vi "test_csm_interface_descp.vi"() -> ()   [LabVIEW 2020]
uses:
  Typedef/Def-Argument Info.ctl
  Create From VI Reference.vi
  Properties/Read User-Defined States.vi
  CSM-Helper.lvclass
panel:
  out "error out":errorcluster
  out "Array 3":cluster{string, "Argument":T1, "Response":T1}[](array[cluster])
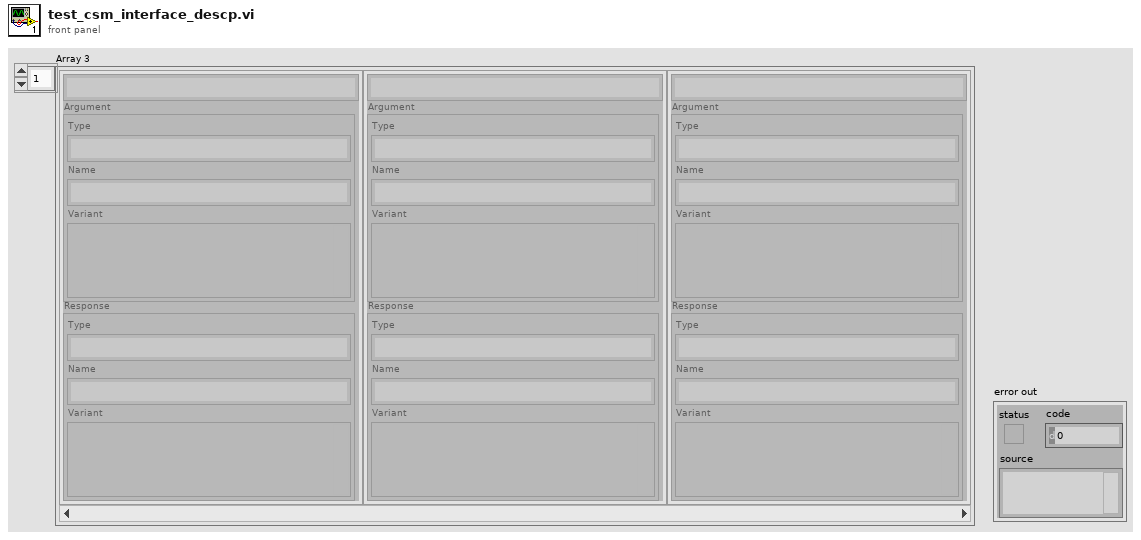
[diagram p1: front panel]
types:
  T1 = typedef "CSM-Helper.lvclass/Def-Argument Info.ctl" = cluster{"Type":string, "Name":string, "Variant":variant}
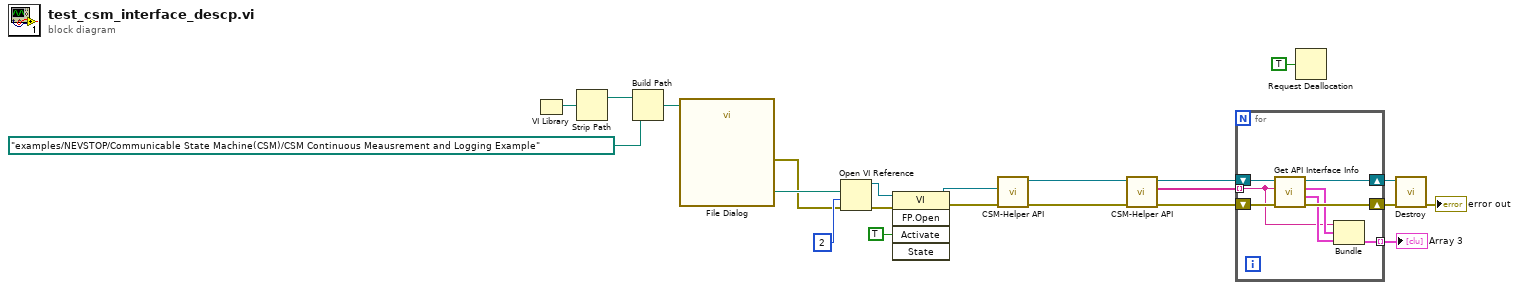
[diagram p0: block diagram]
diagram:
  n1 = VI Library() -> (path=w22:path)
  n2 = Strip Path(path=w22) -> (stripped path=w21:path)  [unwired: 1 out]
  n3 = Build Path(base path=w21, name or relative path=path "examples/NEVSTOP/Communicable State Machine(CSM)/CSM Continuous Meausrement and Logging Example") -> (appended path=w19:path)
  n4 = call "File Dialog"("start path"=w19) -> ("selected path"=w18:path, "error out"=w4:errorcluster)  [unwired: 11 in, 2 out]
  n5 = Open VI Reference(vi path=w18, options=2, error in (no error)=w4) -> (vi reference=w16:refnum<vi>, error out=w15:errorcluster)  [unwired: 3 in]
  n6 = invoke class="VI" method="FP.Open"(reference=w16, error in=w15, "Activate"=TRUE ("Activate?")) -> (reference out=w5:refnum<vi>, error out=w6:errorcluster)  [unwired: 2 in, 3 out]
  n7 = call-poly "CSM-Helper API.vi"("error in (no error)"=w6, "VI"=w5) -> ("error out"=w13:errorcluster, "CSM-Helper.lvclass"=w2:refnum<class "CSM-Helper.lvclass">)  [unwired: 8 in]
  n8 = call-poly "CSM-Helper API.vi"("error in (no error)"=w13, "CSM-Helper in"=w2) -> ("error out"=w12:errorcluster, "Array"=w9:string[], "CSM-Helper out"=w11:refnum<class "CSM-Helper.lvclass">)  [unwired: 7 in]
  n9 = for {
    shift-right: [w27] -> w7
    shift-left: w12 -> [w30]
    shift-right: [w28] -> w8
    shift-left: w11 -> [w29]
    tunnel: w9 -> [w23] mode=indexing
    tunnel: [w24] -> w10 mode=indexing
    n10 = call "Get API Interface Info.vi"("error in (no error)"=w30, "CASE"=w23, "CSM-Helper in"=w29) -> ("error out"=w27:errorcluster, "Response"=w26:T1, "Argument"=w25:T1, "CSM-Helper out"=w28:refnum<class "CSM-Helper.lvclass">)  [unwired: 5 in]
    n11 = Bundle(w23, "Argument"=w25, "Response"=w26) -> (w24:cluster{string, "Argument":T1, "Response":T1})  [unwired: 1 in]
  }
  "Array 3" <- w10
  n12 = Request Deallocation(TRUE ("flag")) -> ()
  n13 = call "Destroy.vi"("error in (no error)"=w7, "CSM-Helper in"=w8) -> ("error out"=→"error out":errorcluster)  [unwired: 8 in, 1 out]
